vi "Disable Selection.vi"(8 "error in (no error)":errorcluster, 10 "Disable?":bool, 11 "Scheduler in":refnum<class "Scheduler.lvclass">=refnum) -> (0 "error out":errorcluster, 3 "Scheduler out":refnum<class "Scheduler.lvclass">)   [LabVIEW 2020, in "CIRCUS_uServices.lvlib" / "Holy Trinity.lvlib" / "Scheduler.lvlib" / "Scheduler.lvclass"]
uses:
  Scheduler.lvclass
  TALOS/TALOS_PPL.lvlibp
  TALOS/TALOS_PPL.lvlibp/Father of all uServices/Father of all uServices/Father of all uServices.lvclass
  C:/Users/marco/Documents/GitHub_Lab/CIRCUS/TALOS/TALOS_PPL.lvlibp/Ancestor/Ancestor/Ancestor.lvclass
  C:/Users/marco/Documents/GitHub_Lab/CIRCUS/TALOS/Actor Framework.lvlibp/1abvi3w/vi.lib/ActorFramework/Actor/Actor.lvclass
  C:/Users/marco/Documents/GitHub_Lab/CIRCUS/TALOS/TALOS_PPL.lvlibp/Father of all uServices/Father of all uServices/Father of all uServices.lvclass
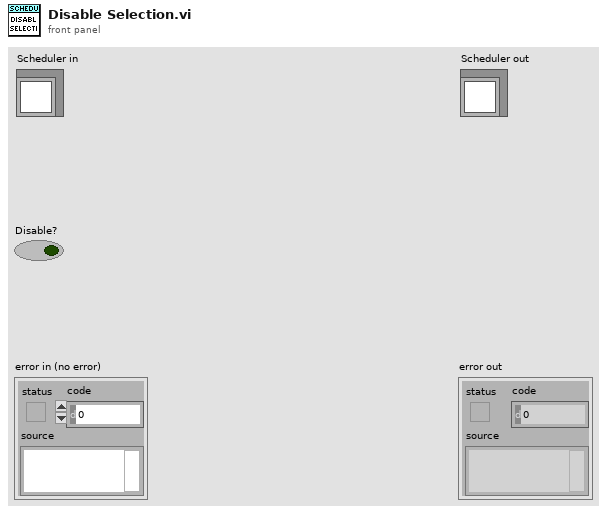
[diagram p1: front panel]
types:
  T1 = enum8{"Enabled", "Disabled", "Disabled and Grayed Out"}
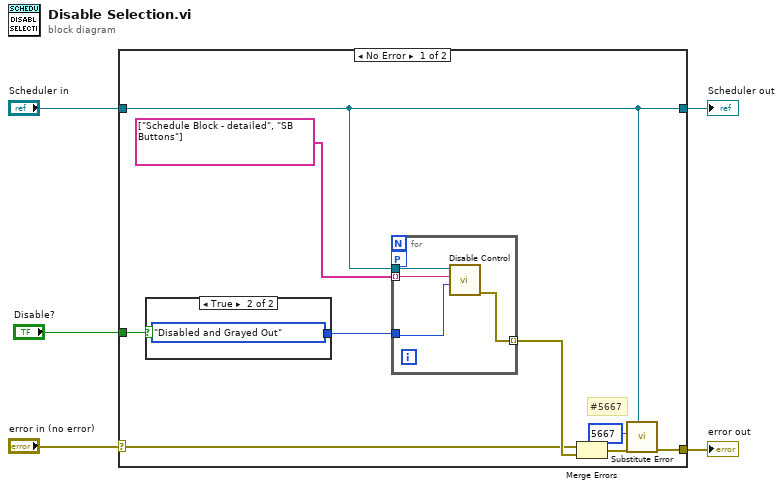
[diagram p0: block diagram]
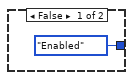
[diagram p2: hidden frame]
diagram:
  n1 = case shown="No Error" "error in (no error)" {
    selector: "error in (no error)" -> [w9 w22]
    tunnel: [w11 w22] -> w4
    tunnel: [w7 w21] -> w2
    tunnel: "Scheduler in" -> [w7 w21]
    tunnel: "Disable?" -> [w14 _]
    frame No Error {
      # "#5667"
      n2 = case shown="True" w14 {
        tunnel: [T1."Enabled" ("Disabled") T1."Disabled and Grayed Out" ("Disabled")] -> w13
        frame False {
        }
        frame True {
        }
      }
      n3 = for {
        tunnel: w13 -> [w18]
        tunnel: string[] ["Schedule Block - detailed", "SB Buttons"] -> [w17] mode=indexing
        tunnel: [w15] -> w10 mode=indexing
        tunnel: w7 -> [w16]
        workers-P: _ -> [_]
        n4 = call "Disable Control.vi"("Disabled"=w18, "FP Item Name"=w17, "Father of all uServices in"=w16) -> ("error out"=w15:errorcluster)  [unwired: 7 in, 1 out]
      }
      n5 = Merge Errors(w9, w10) -> (w8:errorcluster)
      n6 = call "Substitute Error.vi"("LabVIEW Object"=w7, "error in (no error)"=w8, "Error Code"=5667) -> ("error out"=w11:errorcluster)  [unwired: 8 in]
    }
    frame Error {
    }
  }
  "error out" <- w4
  "Scheduler out" <- w2
